vi "DiffVIs.vi"(6 "Title Prefix In":string, 8 "error in":errorcluster, 9 "Picture Save Location":path, 10 "New VI Path":path, 11 "Old VI Path":path) -> (0 "error out":errorcluster, 2 "diff file":path)   [LabVIEW 2015, in "VIDiffScreenshots.lvlib"]
uses:
  VIDiffScreenshots.lvlib
  Utilities/Arguments.ctl
  VIScreenshots.ctl
  ScreenshotInfo.ctl
  Screenshot Type.ctl
  Utilities/FilePaths.ctl
  Utilities/VIDiffUtilities.lvlib
panel:
  out "Description":string
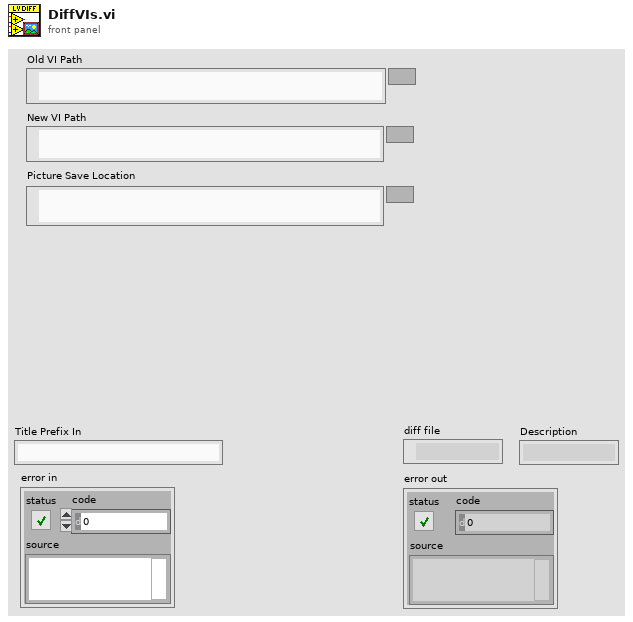
[diagram p1: front panel]
types:
  T1 = typedef "VIDiffScreenshots.lvlib/Screenshot Type.ctl" = enum16{"Unknown", "Front Panel", "Connector Pane", "Block Diagram", "VI Hierarchy"}
  T2 = typedef "VIDiffScreenshots.lvlib/VIScreenshots.ctl" = cluster{"Front Panel Screenshots":T3[], "Block Diagram Screenshots":T3[], "Connector Pane Screenshots":T3[], "VI Hierarchy Screenshots":T3[], "Unknown Screenshots":T3[], "vi reference":refnum<vi>, "File Paths":cluster{"File Path":path, "Container Path":path}, "Name":string}
  T3 = typedef "VIDiffScreenshots.lvlib/ScreenshotInfo.ctl" = cluster{"Screenshot Path":path, "Screenshot Type":T1, "VI Paths":T4}
  T4 = typedef "VIDiffUtilities.lvlib/FilePaths.ctl" = cluster{"File Path":path, "Container Path":path}
  T5 = typedef "VIDiffUtilities.lvlib/Arguments.ctl" = cluster{"VI 1 Path":path, "VI 2 Path":path, "Picture Save Location":path, "Screenshot Title":string}
  T6 = typedef "VIDiffUtilities.lvlib/Output Folders.ctl" = cluster{"combined":path, "vi1shots":path, "vi2shots":path, "Picture Save Location":path}
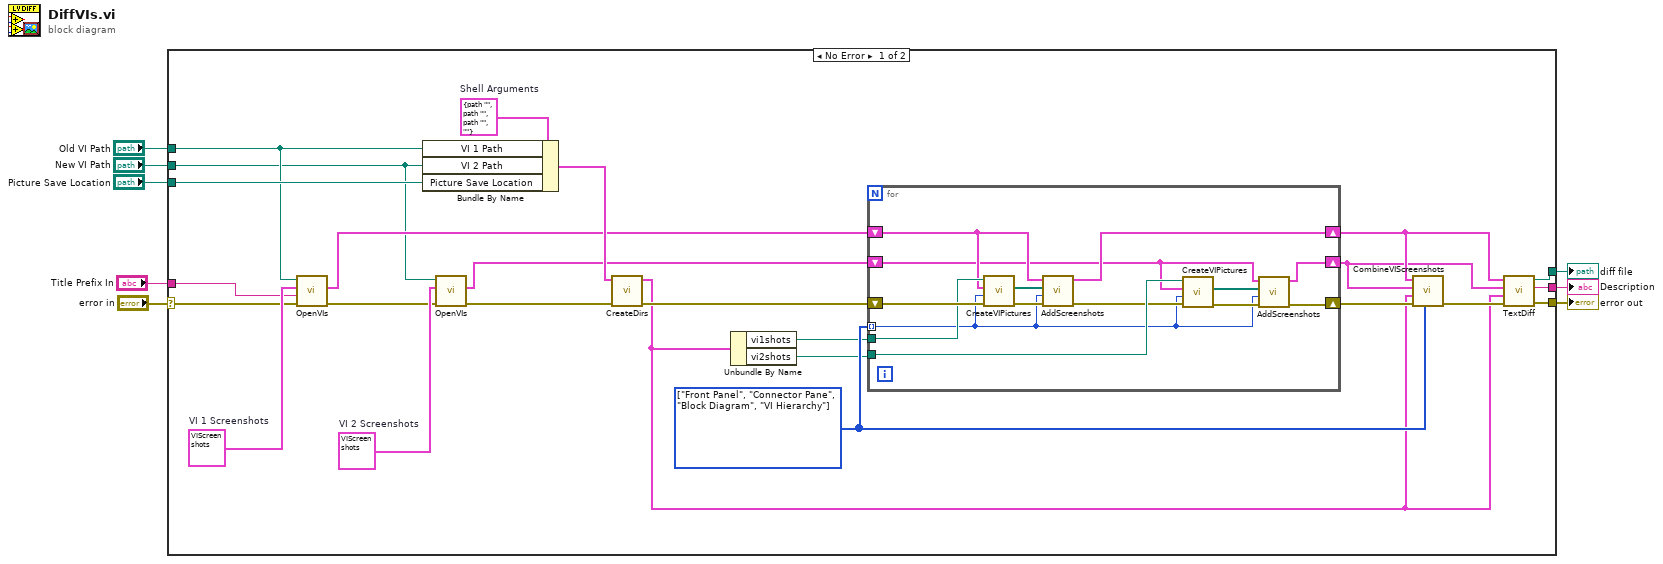
[diagram p0: block diagram]
diagram:
  n1 = case shown="No Error" "error in" {
    selector: "error in" -> [w9 w48]
    tunnel: [w32 _] -> w8
    tunnel: "Picture Save Location" -> [w31 _]
    tunnel: [w24 _] -> w6
    tunnel: [w17 w48] -> w5
    tunnel: "Old VI Path" -> [w16 _]
    tunnel: "New VI Path" -> [w13 _]
    tunnel: "Title Prefix In" -> [w10 _]
    frame No Error {
      w27 = T1[] [enum."Front Panel", enum."Connector Pane", enum."Block Diagram", enum."VI Hierarchy"] items=["Unknown", "Front Panel", "Connector Pane", "Block Diagram", "VI Hierarchy"]
      w14 = T2 {"Front Panel Screenshots"=[], "Block Diagram Screenshots"=[], "Connector Pane Screenshots"=[], "VI Hierarchy Screenshots"=[], "Unknown Screenshots"=[], "vi reference"=refnum, "File Paths"={"File Path"=path "", "Container Path"=path ""}, "Name"=""}  # VI 2 Screenshots
      w29 = T2 {"Front Panel Screenshots"=[], "Block Diagram Screenshots"=[], "Connector Pane Screenshots"=[], "VI Hierarchy Screenshots"=[], "Unknown Screenshots"=[], "vi reference"=refnum, "File Paths"={"File Path"=path "", "Container Path"=path ""}, "Name"=""}  # VI 1 Screenshots
      w33 = T5 {"VI 1 Path"=path "", "VI 2 Path"=path "", "Picture Save Location"=path "", "Screenshot Title"=""}  # Shell Arguments
      n2 = call "OpenVIs.vi"("error in (no error)"=w9, "Title Prefix In"=w10, "VI Screenshots"=w29, "VI Path"=w16) -> ("error out"=w11:errorcluster, "VI Screenshots out"=w22:T2)  [unwired: 6 in]
      n3 = Bundle By Name(cluster=w33, "VI 1 Path"=w16, "VI 2 Path"=w13, "Picture Save Location"=w31) -> (w30:T5)
      n4 = call "OpenVIs.vi"("error in (no error)"=w11, "VI Screenshots"=w14, "VI Path"=w13) -> ("error out"=w15:errorcluster, "VI Screenshots out"=w12:T2)  [unwired: 7 in]
      n5 = call "CreateDirs.vi"("error in (no error)"=w15, "Shell Arguments"=w30) -> ("error out"=w21:errorcluster, "Output Folders"=w18:T6)  [unwired: 8 in]
      n6 = Unbundle By Name(w18) -> ("vi1shots"=w26:path, "vi2shots"=w25:path)
      n7 = for {
        tunnel: w27 -> [w34] mode=indexing
        shift-right: [w42] -> w28
        shift-left: w21 -> [w47]
        tunnel: w26 -> [w46]
        tunnel: w25 -> [w45]
        shift-right: [w41] -> w20
        shift-left: w22 -> [w39]
        shift-right: [w40] -> w19
        shift-left: w12 -> [w38]
        n8 = call "CreateVIPictures.vi"("error in (no error)"=w47, "Capture Target"=w34, "VI 1 Screenshots"=w39, "Picture Save Location"=w46) -> ("error out"=w37:errorcluster, "Screenshot Files"=w44:path[])  [unwired: 6 in]
        n9 = call "AddScreenshots.vi"("error in (no error)"=w37, "Screenshot Type"=w34, "Screenshot Paths"=w44, "VI Screenshots In"=w39) -> ("error out"=w36:errorcluster, "VI Screenshots Out"=w41:T2)  [unwired: 6 in]
        n10 = call "CreateVIPictures.vi"("error in (no error)"=w36, "Capture Target"=w34, "VI 1 Screenshots"=w38, "Picture Save Location"=w45) -> ("error out"=w35:errorcluster, "Screenshot Files"=w43:path[])  [unwired: 6 in]
        n11 = call "AddScreenshots.vi"("error in (no error)"=w35, "Screenshot Type"=w34, "Screenshot Paths"=w43, "VI Screenshots In"=w38) -> ("error out"=w42:errorcluster, "VI Screenshots Out"=w40:T2)  [unwired: 6 in]
      }
      n12 = call "CombineVIScreenshots.vi"("Image Types"=w27, "error in (no error)"=w28, "Output Folders"=w18, "NewVI Screenshots in"=w19, "OldVI Screenshots in"=w20) -> ("error out"=w23:errorcluster)  [unwired: 6 in]
      n13 = call "TextDiff.vi"("error in (no error)"=w23, "Output Folders"=w18, "VI 2 Screenshots in"=w19, "VI 1 Screenshots in"=w20) -> ("error out"=w17:errorcluster, "Description"=w24:string, "appended path"=w32:path)  [unwired: 5 in]
    }
    frame Error {
    }
  }
  "diff file" <- w8
  "Description" <- w6
  "error out" <- w5
